vi "Converge.vi"   [LabVIEW 2017]
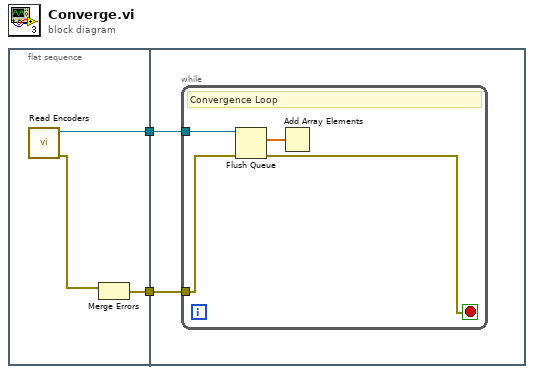
[diagram p0: block diagram]
diagram:
  n1 = flat-sequence {
    tunnel: [w4] -> w2
    tunnel: [w3] -> w1
    tunnel: w2 -> [w7]
    tunnel: w1 -> [w6]
    frame #0 {
      n2 = call "Read Encoders.vi"() -> ("error out"=w5:errorcluster, "queue out"=w3:refnum<queue>)  [unwired: 10 in]
      n3 = Merge Errors(w5) -> (w4:errorcluster)  [unwired: 1 in]
    }
    frame #1 {
      n4 = while {
        tunnel: w7 -> [w9]
        tunnel: w6 -> [w11]
        stop <- w8 stop-if-true
        # "Convergence Loop"
        n5 = Flush Queue(queue=w11, error in (no error)=w9) -> (remaining elements=w10:dbl[], error out=w8:errorcluster)  [unwired: 1 out]
        n6 = Add Array Elements(numeric array=w10) -> ()  [unwired: 1 out]
      }
    }
  }
